vi "testingauto2.vi"() -> ()   [LabVIEW 2014]
uses:
  <vilib>/vision/NI_Vision_Development_Module.lvlib
  <instrlib>/KD Scientific 2XX Series/KD Scientific 2XX Series.lvlib
panel:
  in  "stop 3":bool
  in  "Initial Pressure":dbl[](array[numeric])
  in  "Number of Cycles":i32
  in  "Min Pressure":dbl
  in  "Max Pressure":dbl
  out "Status":T1
  in  "stop 2":bool
  out "Delivered Volume":dbl
  out "Units":string
  in  "Baud Rate (9600)":u32(ring)=9600 items=["300"=300, "1200"=1200, "2400"=2400, "4800"=4800, "9600"=9600]
  in  "Withdrawal Settings":T2={"Flow Rate (5)"=5.0, "Volume (10)"=10.0, "Volume Units (ml)"=enum."milliliters (ml)", "Rate Units (ml/min.)"=enum."milliliters per minute (ml/min.)"} {"Volume (10)" format="%#.3g"}
  in  "Diameter (8.75 mm)":dbl=8.75
  in  "Infusion Settings":T2={"Flow Rate (5)"=5.0, "Volume (10)"=10.0, "Volume Units (ml)"=enum."milliliters (ml)", "Rate Units (ml/min.)"=enum."milliliters per minute (ml/min.)"}
  in  "Address (0)":i32 format="%0.0f"
  in  "error in (no error)":errorcluster
  in  "VISA resource name":refnum<visa-resource-name>="COM1"
  in  "stop":bool
  out "Image":T3(plugin-control)
  out "Particle Measurements (Pixels) (Particle Analysis 1)":dbl[][](array[numeric]) format="%.2f"
  out "subarray":dbl[](array[numeric])
  out "The diameter":dbl[](array[numeric])
  in  "stop (F)":bool
  out "Data from Transducer":dynamicdata(graph) caption="Voltage from Transducer V"
  out "Voltage from pressure transducer":dbl[](array[numeric])
  out "Pressure mm Hg":dbl[](graph)
  in  "Calibration factor":dbl[](array[numeric])
  in  "Zero Error":dbl[](array[numeric])
  out "pressure mm Hg":dbl[](array[numeric])
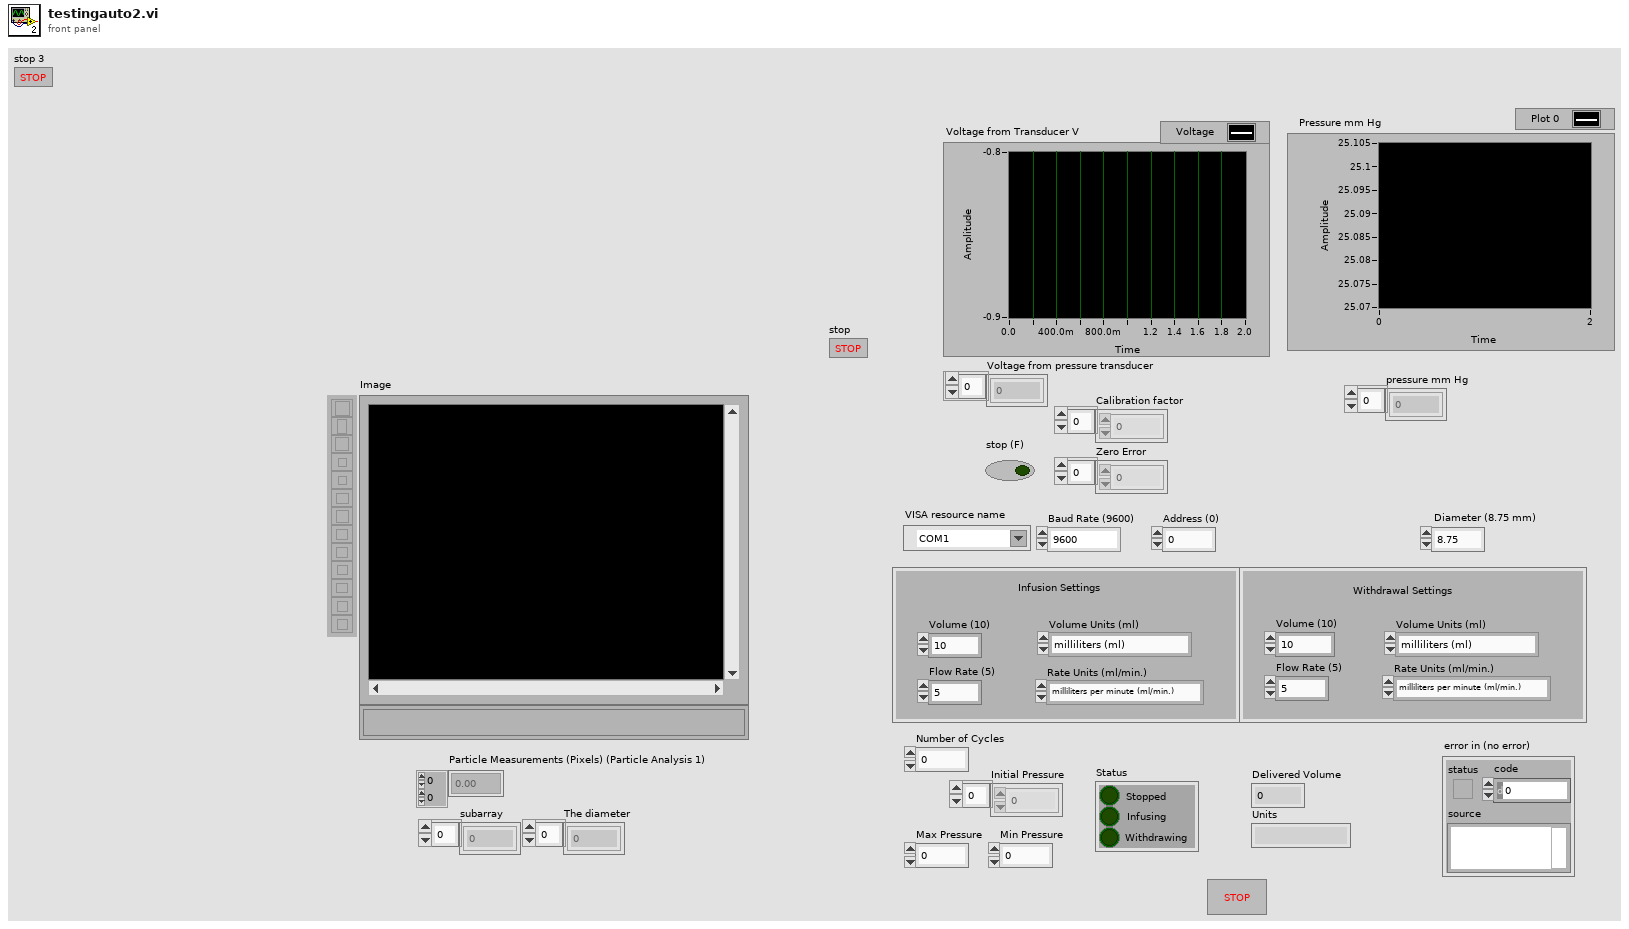
[diagram p1: front panel]
types:
  T1 = cluster{"Stopped":bool, "Infusing":bool, "Withdrawing":bool}
  T2 = cluster{"Flow Rate (5)":dbl, "Volume (10)":dbl, "Volume Units (ml)":enum16{"milliliters (ml)", "microliters (ul)"}, "Rate Units (ml/min.)":enum16{"milliliters per minute (ml/min.)", "milliliters per hour (ml/hr.)", "microliters per minute (ul/min.)", "microliters per hour (ul/hr.)"}}
  T3 = typedef "IMAQ Image.ctl" = refnum<image>
  T4 = typedef "Board Id" = u8
  T5 = typedef "ROI Descriptor" = cluster{"Global Rectangle":i32[], "Contours":cluster{"ID":enum32{"External", "Internal"}, "Type":u32, "Coordinates":i32[]}[]}
  T6 = enum16{"milliliters per minute (ml/min.)", "milliliters per hour (ml/hr.)", "microliters per minute (ul/min.)", "microliters per hour (ul/hr.)"}
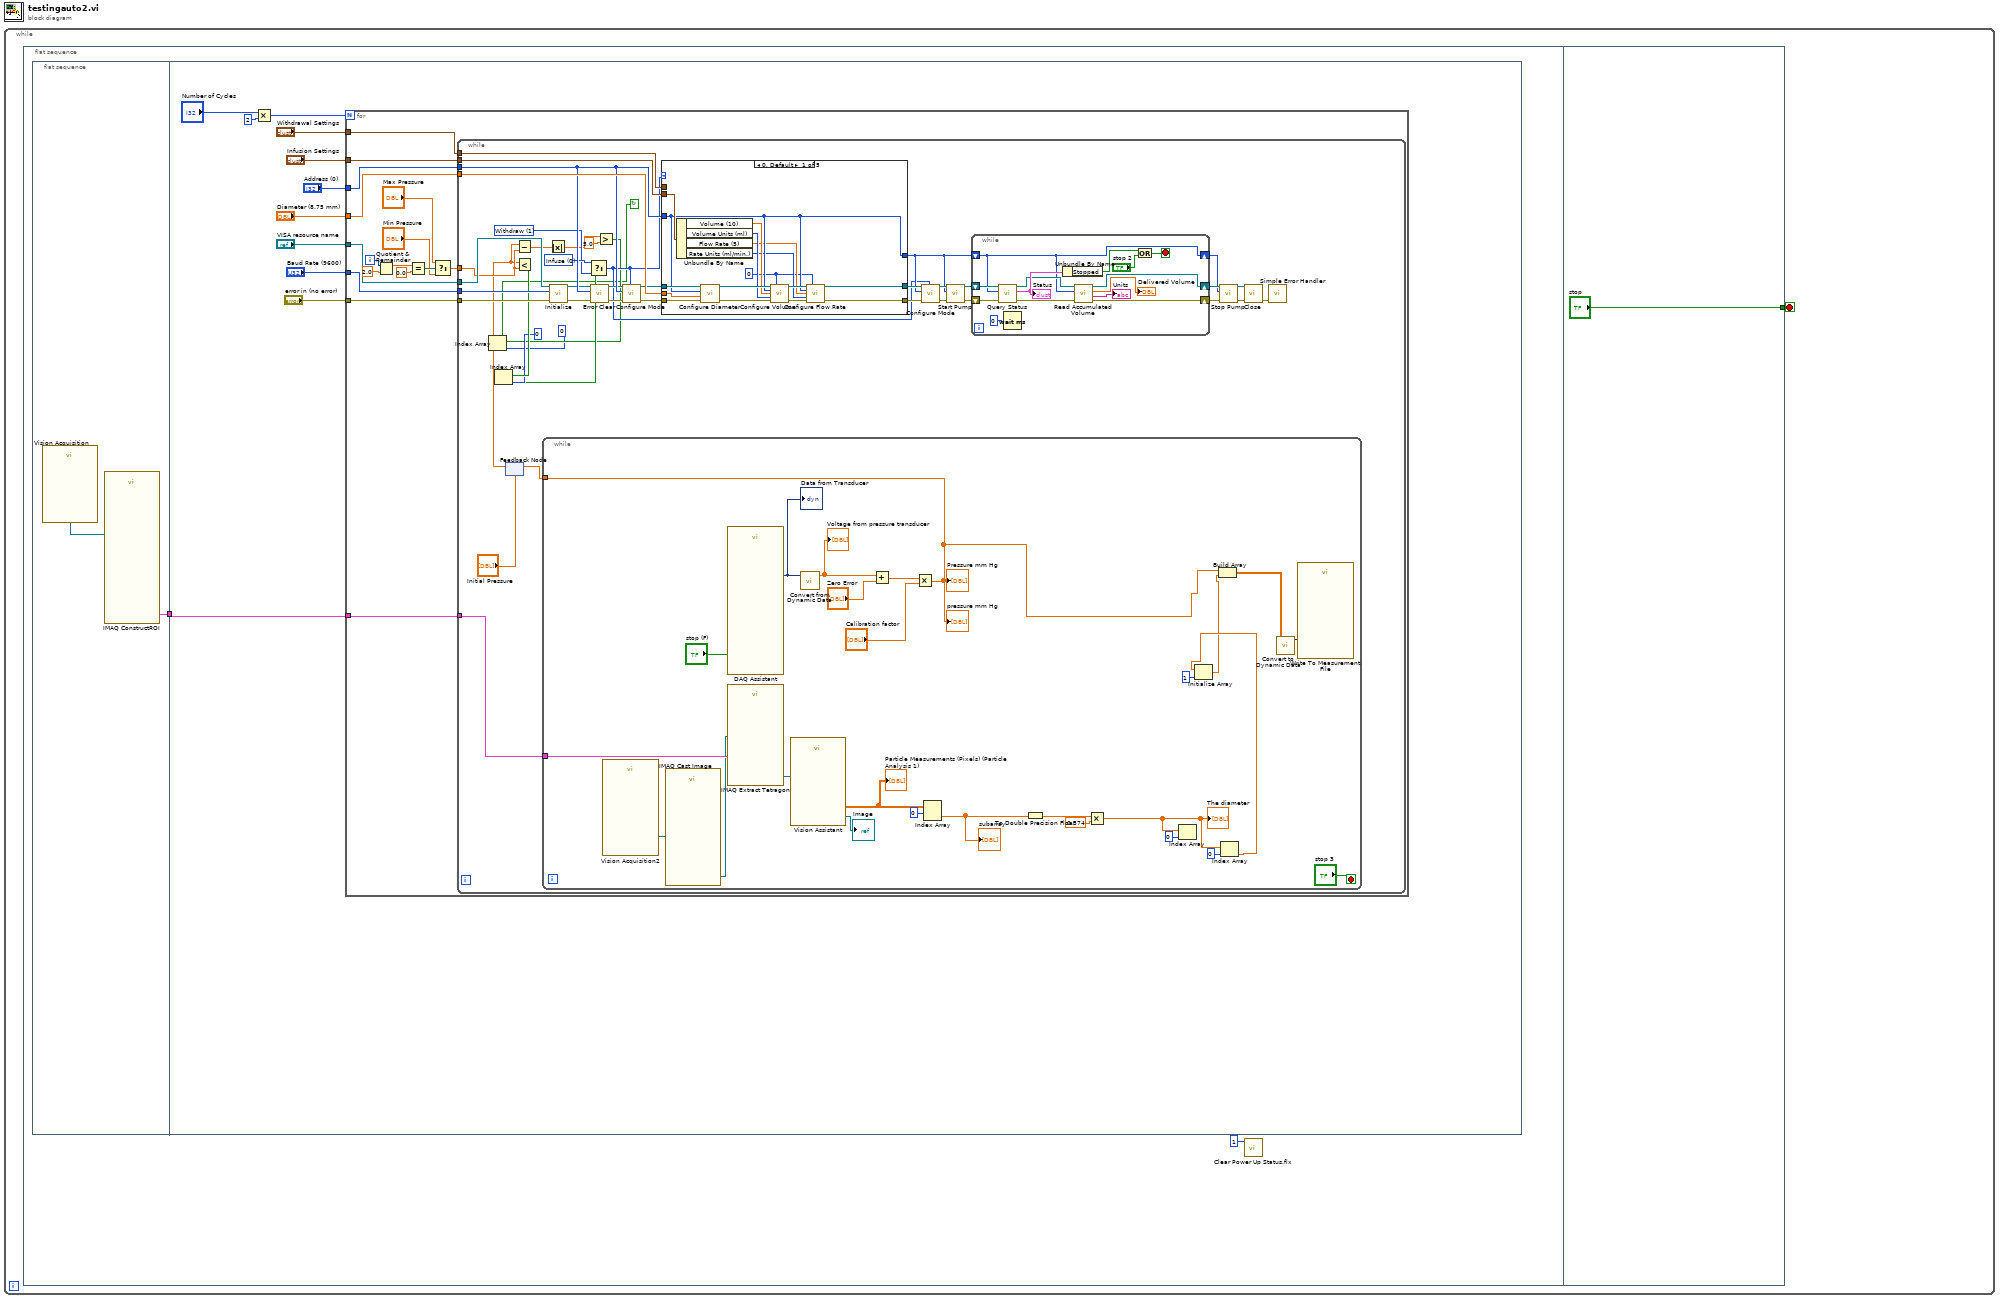
[diagram p0: block diagram]
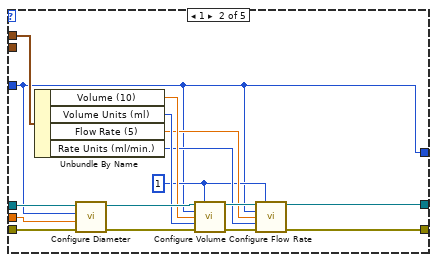
[diagram p2: hidden frame]
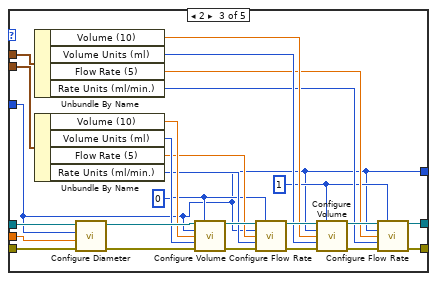
[diagram p3: hidden frame]
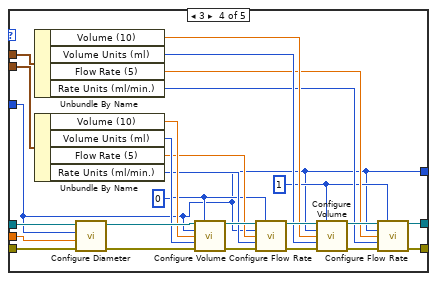
[diagram p4: hidden frame]
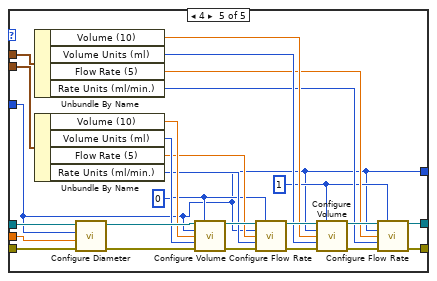
[diagram p5: hidden frame]
diagram:
  n1 = while {
    stop <- w1 stop-if-true
    n2 = flat-sequence {
      tunnel: ["stop"] -> w1
      frame #0 {
        n3 = flat-sequence {
          tunnel: [w4] -> w3
          tunnel: w3 -> [w6]
          frame #0 {
            n4 = call "Vision Acquisition"() -> ("Image Out"=w5:T3)  [unwired: 26 in, 1 out]
            n5 = call "IMAQ ConstructROI"("Image"=w5) -> ("ROI Descriptor Out"=w4:T5)  [unwired: 7 in, 3 out]
          }
          frame #1 {
            n6 = Multiply(x="Number of Cycles", y=2) -> (x*y=w16:i32)
            n7 = for {
              N: w16 -> [_]
              tunnel: "VISA resource name" -> [w32]
              tunnel: "error in (no error)" -> [w31]
              tunnel: "Infusion Settings" -> [w30]
              tunnel: "Withdrawal Settings" -> [w29]
              tunnel: "Diameter (8.75 mm)" -> [w28]
              tunnel: "Baud Rate (9600)" -> [w27]
              tunnel: "Address (0)" -> [w26]
              tunnel: w6 -> [w17]
              i -> [w24]
              n8 = Quotient & Remainder(x=w24, y=2.0) -> (x-y*floor(x/y)=w22:dbl)  [unwired: 1 out]
              n9 = Equal?(x=w22, y=0.0) -> (x = y?=w21:bool)
              n10 = Select(t="Max Pressure", s=w21, f="Min Pressure") -> (s? t:f=w18:dbl)
              n11 = while {
                tunnel: w32 -> [w75]
                tunnel: w31 -> [w74]
                tunnel: w30 -> [w73]
                tunnel: w29 -> [w72]
                tunnel: w28 -> [w71]
                tunnel: w27 -> [w70]
                tunnel: w26 -> [w69]
                tunnel: w18 -> [w46]
                tunnel: w17 -> [w36]
                stop <- w37 continue-if-true
                w48 = u16 1 items=["Withdraw"=1]
                w49 = u16 0 items=["Infuse"] ("Mode (infuse)")
                n12 = feedback #1("Initial Pressure") -> (w34:dbl[])
                n13 = Subtract(x=w34, y=w46) -> (x-y=w45:dbl[])
                n14 = Less?(x=w34, y=w46) -> (x < y?=w42:bool[])
                n15 = Index Array(array=w42, index=0) -> (element=w40:bool)
                n16 = while {
                  tunnel: w36 -> [w84]
                  tunnel: [w81] -> w35
                  stop <- "stop 3" stop-if-true
                  n17 = call "Vision Acquisition2"() -> ("Image Out"=w93:T3)  [unwired: 25 in, 2 out]
                  n18 = call "IMAQ Cast Image"("Image Src"=w93) -> ("Image Dst Out"=w83:T3)  [unwired: 9 in, 1 out]
                  n19 = call "DAQ Assistant"("stop (F)"="stop (F)") -> ("data"=w96:dynamicdata)  [unwired: 15 in, 3 out]
                  "Data from Transducer" <- w96
                  n20 = call-poly "IMAQ Extract Tetragon"("ROI Descriptor"=w84, "Image Src"=w83) -> ("Image Dst Out"=w86:T3)  [unwired: 8 in, 1 out]
                  n21 = call "Vision Assistant"("Image In"=w86) -> ("Image Out"=→"Image":T3, "Particle Measurements (Pixels) (Particle Analysis 1)"=w87:dbl[][])  [unwired: 23 in, 2 out]
                  "Particle Measurements (Pixels) (Particle Analysis 1)" <- w87
                  n22 = call "Convert from Dynamic Data"("Dynamic Data Type"=w96) -> ("Array"=w99:dbl[])  [unwired: 3 in]
                  "Voltage from pressure transducer" <- w99
                  n23 = Add(x=w99, y="Zero Error") -> (x+y=w97:dbl[])
                  n24 = Multiply(x=w97, y="Calibration factor") -> (x*y=w81:dbl[])
                  "Pressure mm Hg" <- w81
                  "pressure mm Hg" <- w81
                  n25 = Index Array(array=w87, index (row)=0) -> (element=w89:dbl[])  [unwired: 1 in]
                  "subarray" <- w89
                  n26 = To Double Precision Float(number=w89) -> (double precision float=w90:dbl[])
                  n27 = Multiply(x=w90, y=0.374) -> (x*y=w95:dbl[])
                  "The diameter" <- w95
                  n28 = Index Array(array=w95, index=0) -> ()  [unwired: 1 out]
                  n29 = Index Array(array=w95, index=0) -> (element=w80:dbl)
                  n30 = Initialize Array(w80, 1 ("dimension size")) -> (w79:dbl[])
                  n31 = Build Array(w81, w79) -> (w78:dbl[][])
                  n32 = call "Convert to Dynamic Data"("2D Array"=w78) -> ("Dynamic Data Type"=w77:dynamicdata)  [unwired: 3 in]
                  n33 = call "Write To Measurement File"("Signals"=w77) -> ()  [unwired: 16 in, 3 out]
                }
                n34 = feedback-in #1(w35) -> ()
                n35 = Absolute Value(x=w45) -> (abs(x)=w44:dbl[])
                n36 = call <instrlib>:"Initialize.vi"("error in (no error)"=w74, "Baud Rate (9600)"=w70, "VISA resource name"=w75) -> ("error out"=w51:errorcluster, "VISA resource name out"=w50:refnum<visa-resource-name>)  [unwired: 7 in]
                n37 = Select(t=w49, s=w40, f=w48) -> (s? t:f=w47:u16)
                n38 = call <instrlib>:"Error Clear.vi"("error in (no error)"=w51, "Address (0)"=w69, "VISA resource name"=w50) -> ("error out"=w52:errorcluster, "VISA resource name out"=w53:refnum<visa-resource-name>)  [unwired: 6 in, 1 out]
                n39 = Greater?(x=w44, y=5.0) -> (0:w39:bool[])
                n40 = Index Array(array=w39, index=0) -> (element=w37:bool)
                n41 = call <instrlib>:"Configure Mode.vi"("Mode (infuse)"=w47, "error in (no error)"=w52, "Address (0)"=w69, "VISA resource name"=w53) -> ("error out"=w55:errorcluster, "VISA resource name out"=w54:refnum<visa-resource-name>)  [unwired: 6 in]
                n42 = case shown="0, Default" w47 {
                  tunnel: w73 -> [w111 _ w159 w185 w211]
                  tunnel: w72 -> [_ w133 w158 w184 w210]
                  tunnel: w54 -> [w117 w132 w157 w183 w209]
                  tunnel: w55 -> [w116 w128 w156 w182 w208]
                  tunnel: w71 -> [w110 w124 w139 w165 w191]
                  tunnel: [w109 w118 w134 w160 w186] -> w56
                  tunnel: w69 -> [w109 w118 w134 w160 w186]
                  tunnel: [w104 w129 w136 w162 w188] -> w60
                  tunnel: [w103 w125 w135 w161 w187] -> w59
                  frame 0, Default {
                    w102 = 0
                    n43 = Unbundle By Name(w111) -> ("Volume (10)"=w108:dbl, "Volume Units (ml)"=w107:enum16{"milliliters (ml)", "microliters (ul)"}, "Flow Rate (5)"=w106:dbl, "Rate Units (ml/min.)"=w105:T6)
                    n44 = call <instrlib>:"Configure Diameter.vi"("error in (no error)"=w116, "Diameter (8.75 mm)"=w110, "Address (0)"=w109, "VISA resource name"=w117) -> ("error out"=w114:errorcluster, "VISA resource name out"=w115:refnum<visa-resource-name>)  [unwired: 6 in]
                    n45 = call <instrlib>:"Configure Volume.vi"("VISA resource name"=w115, "Mode (infuse)"=w102, "Address (0)"=w109, "Volume (100)"=w108, "Units (0: milliliters)"=w107, "error in (no error)"=w114) -> ("VISA resource name out"=w113:refnum<visa-resource-name>, "error out"=w112:errorcluster)  [unwired: 8 in]
                    n46 = call <instrlib>:"Configure Flow Rate.vi"("VISA resource name"=w113, "Mode (infuse)"=w102, "Address (0)"=w109, "Flow Rate (5)"=w106, "Units (0: milliliters per minute)"=w105, "error in (no error)"=w112) -> ("VISA resource name out"=w104:refnum<visa-resource-name>, "error out"=w103:errorcluster)  [unwired: 8 in]
                  }
                  frame 1 {
                    w119 = 1
                    n47 = Unbundle By Name(w133) -> ("Volume (10)"=w123:dbl, "Volume Units (ml)"=w122:enum16{"milliliters (ml)", "microliters (ul)"}, "Flow Rate (5)"=w121:dbl, "Rate Units (ml/min.)"=w120:T6)
                    n48 = call <instrlib>:"Configure Diameter.vi"("error in (no error)"=w128, "Diameter (8.75 mm)"=w124, "Address (0)"=w118, "VISA resource name"=w132) -> ("error out"=w127:errorcluster, "VISA resource name out"=w131:refnum<visa-resource-name>)  [unwired: 6 in]
                    n49 = call <instrlib>:"Configure Volume.vi"("VISA resource name"=w131, "Mode (infuse)"=w119, "Address (0)"=w118, "Volume (100)"=w123, "Units (0: milliliters)"=w122, "error in (no error)"=w127) -> ("VISA resource name out"=w130:refnum<visa-resource-name>, "error out"=w126:errorcluster)  [unwired: 8 in]
                    n50 = call <instrlib>:"Configure Flow Rate.vi"("VISA resource name"=w130, "Mode (infuse)"=w119, "Address (0)"=w118, "Flow Rate (5)"=w121, "Units (0: milliliters per minute)"=w120, "error in (no error)"=w126) -> ("VISA resource name out"=w129:refnum<visa-resource-name>, "error out"=w125:errorcluster)  [unwired: 8 in]
                  }
                  frame 2 {
                    w137 = 1
                    w138 = 0
                    n51 = Unbundle By Name(w158) -> ("Volume (10)"=w143:dbl, "Volume Units (ml)"=w142:enum16{"milliliters (ml)", "microliters (ul)"}, "Flow Rate (5)"=w141:dbl, "Rate Units (ml/min.)"=w140:T6)
                    n52 = Unbundle By Name(w159) -> ("Volume (10)"=w147:dbl, "Volume Units (ml)"=w146:enum16{"milliliters (ml)", "microliters (ul)"}, "Flow Rate (5)"=w145:dbl, "Rate Units (ml/min.)"=w144:T6)
                    n53 = call <instrlib>:"Configure Diameter.vi"("error in (no error)"=w156, "Diameter (8.75 mm)"=w139, "Address (0)"=w134, "VISA resource name"=w157) -> ("error out"=w151:errorcluster, "VISA resource name out"=w155:refnum<visa-resource-name>)  [unwired: 6 in]
                    n54 = call <instrlib>:"Configure Volume.vi"("VISA resource name"=w155, "Mode (infuse)"=w138, "Address (0)"=w134, "Volume (100)"=w147, "Units (0: milliliters)"=w146, "error in (no error)"=w151) -> ("VISA resource name out"=w154:refnum<visa-resource-name>, "error out"=w150:errorcluster)  [unwired: 8 in]
                    n55 = call <instrlib>:"Configure Flow Rate.vi"("VISA resource name"=w154, "Mode (infuse)"=w138, "Address (0)"=w134, "Flow Rate (5)"=w145, "Units (0: milliliters per minute)"=w144, "error in (no error)"=w150) -> ("VISA resource name out"=w153:refnum<visa-resource-name>, "error out"=w149:errorcluster)  [unwired: 8 in]
                    n56 = call <instrlib>:"Configure Volume.vi"("VISA resource name"=w153, "Mode (infuse)"=w137, "Address (0)"=w134, "Volume (100)"=w143, "Units (0: milliliters)"=w142, "error in (no error)"=w149) -> ("VISA resource name out"=w152:refnum<visa-resource-name>, "error out"=w148:errorcluster)  [unwired: 8 in]
                    n57 = call <instrlib>:"Configure Flow Rate.vi"("VISA resource name"=w152, "Mode (infuse)"=w137, "Address (0)"=w134, "Flow Rate (5)"=w141, "Units (0: milliliters per minute)"=w140, "error in (no error)"=w148) -> ("VISA resource name out"=w136:refnum<visa-resource-name>, "error out"=w135:errorcluster)  [unwired: 8 in]
                  }
                  frame 3 {
                    w163 = 1
                    w164 = 0
                    n58 = Unbundle By Name(w184) -> ("Volume (10)"=w169:dbl, "Volume Units (ml)"=w168:enum16{"milliliters (ml)", "microliters (ul)"}, "Flow Rate (5)"=w167:dbl, "Rate Units (ml/min.)"=w166:T6)
                    n59 = Unbundle By Name(w185) -> ("Volume (10)"=w173:dbl, "Volume Units (ml)"=w172:enum16{"milliliters (ml)", "microliters (ul)"}, "Flow Rate (5)"=w171:dbl, "Rate Units (ml/min.)"=w170:T6)
                    n60 = call <instrlib>:"Configure Diameter.vi"("error in (no error)"=w182, "Diameter (8.75 mm)"=w165, "Address (0)"=w160, "VISA resource name"=w183) -> ("error out"=w177:errorcluster, "VISA resource name out"=w181:refnum<visa-resource-name>)  [unwired: 6 in]
                    n61 = call <instrlib>:"Configure Volume.vi"("VISA resource name"=w181, "Mode (infuse)"=w164, "Address (0)"=w160, "Volume (100)"=w173, "Units (0: milliliters)"=w172, "error in (no error)"=w177) -> ("VISA resource name out"=w180:refnum<visa-resource-name>, "error out"=w176:errorcluster)  [unwired: 8 in]
                    n62 = call <instrlib>:"Configure Flow Rate.vi"("VISA resource name"=w180, "Mode (infuse)"=w164, "Address (0)"=w160, "Flow Rate (5)"=w171, "Units (0: milliliters per minute)"=w170, "error in (no error)"=w176) -> ("VISA resource name out"=w179:refnum<visa-resource-name>, "error out"=w175:errorcluster)  [unwired: 8 in]
                    n63 = call <instrlib>:"Configure Volume.vi"("VISA resource name"=w179, "Mode (infuse)"=w163, "Address (0)"=w160, "Volume (100)"=w169, "Units (0: milliliters)"=w168, "error in (no error)"=w175) -> ("VISA resource name out"=w178:refnum<visa-resource-name>, "error out"=w174:errorcluster)  [unwired: 8 in]
                    n64 = call <instrlib>:"Configure Flow Rate.vi"("VISA resource name"=w178, "Mode (infuse)"=w163, "Address (0)"=w160, "Flow Rate (5)"=w167, "Units (0: milliliters per minute)"=w166, "error in (no error)"=w174) -> ("VISA resource name out"=w162:refnum<visa-resource-name>, "error out"=w161:errorcluster)  [unwired: 8 in]
                  }
                  frame 4 {
                    w189 = 1
                    w190 = 0
                    n65 = Unbundle By Name(w210) -> ("Volume (10)"=w195:dbl, "Volume Units (ml)"=w194:enum16{"milliliters (ml)", "microliters (ul)"}, "Flow Rate (5)"=w193:dbl, "Rate Units (ml/min.)"=w192:T6)
                    n66 = Unbundle By Name(w211) -> ("Volume (10)"=w199:dbl, "Volume Units (ml)"=w198:enum16{"milliliters (ml)", "microliters (ul)"}, "Flow Rate (5)"=w197:dbl, "Rate Units (ml/min.)"=w196:T6)
                    n67 = call <instrlib>:"Configure Diameter.vi"("error in (no error)"=w208, "Diameter (8.75 mm)"=w191, "Address (0)"=w186, "VISA resource name"=w209) -> ("error out"=w203:errorcluster, "VISA resource name out"=w207:refnum<visa-resource-name>)  [unwired: 6 in]
                    n68 = call <instrlib>:"Configure Volume.vi"("VISA resource name"=w207, "Mode (infuse)"=w190, "Address (0)"=w186, "Volume (100)"=w199, "Units (0: milliliters)"=w198, "error in (no error)"=w203) -> ("VISA resource name out"=w206:refnum<visa-resource-name>, "error out"=w202:errorcluster)  [unwired: 8 in]
                    n69 = call <instrlib>:"Configure Flow Rate.vi"("VISA resource name"=w206, "Mode (infuse)"=w190, "Address (0)"=w186, "Flow Rate (5)"=w197, "Units (0: milliliters per minute)"=w196, "error in (no error)"=w202) -> ("VISA resource name out"=w205:refnum<visa-resource-name>, "error out"=w201:errorcluster)  [unwired: 8 in]
                    n70 = call <instrlib>:"Configure Volume.vi"("VISA resource name"=w205, "Mode (infuse)"=w189, "Address (0)"=w186, "Volume (100)"=w195, "Units (0: milliliters)"=w194, "error in (no error)"=w201) -> ("VISA resource name out"=w204:refnum<visa-resource-name>, "error out"=w200:errorcluster)  [unwired: 8 in]
                    n71 = call <instrlib>:"Configure Flow Rate.vi"("VISA resource name"=w204, "Mode (infuse)"=w189, "Address (0)"=w186, "Flow Rate (5)"=w193, "Units (0: milliliters per minute)"=w192, "error in (no error)"=w200) -> ("VISA resource name out"=w188:refnum<visa-resource-name>, "error out"=w187:errorcluster)  [unwired: 8 in]
                  }
                }
                n72 = call <instrlib>:"Configure Mode.vi"("Mode (infuse)"=w47, "error in (no error)"=w59, "Address (0)"=w56, "VISA resource name"=w60) -> ("error out"=w57:errorcluster, "VISA resource name out"=w58:refnum<visa-resource-name>)  [unwired: 6 in]
                n73 = call <instrlib>:"Start Pump.vi"("error in (no error)"=w57, "Address (0)"=w56, "VISA resource name"=w58) -> ("error out"=w67:errorcluster, "VISA resource name out"=w68:refnum<visa-resource-name>)  [unwired: 7 in]
                n74 = while {
                  shift-right: [w214] -> w64
                  shift-left: w56 -> [w214]
                  shift-right: [w216] -> w66
                  shift-left: w68 -> [w222]
                  shift-right: [w215] -> w65
                  shift-left: w67 -> [w223]
                  stop <- w220 stop-if-true
                  n75 = call <instrlib>:"Query Status.vi"("error in (no error)"=w223, "Address (0)"=w214, "VISA resource name"=w222) -> ("error out"=w225:errorcluster, "Status"=w221:T1, "VISA resource name out"=w217:refnum<visa-resource-name>)  [unwired: 6 in]
                  "Status" <- w221
                  n76 = Wait (ms)(milliseconds to wait=u32 0) -> ()  [unwired: 1 out]
                  n77 = Unbundle By Name(w221) -> ("Stopped"=w219:bool)
                  n78 = call <instrlib>:"Read Accumulated Volume.vi"("error in (no error)"=w225, "Address (0)"=w214, "VISA resource name"=w217) -> ("error out"=w215:errorcluster, "Units"=→"Units":string, "Delivered Volume"=→"Delivered Volume":dbl, "VISA resource name out"=w216:refnum<visa-resource-name>)  [unwired: 5 in]
                  n79 = Or(x=w219, y="stop 2") -> (x .or. y?=w220:bool)
                }
                n80 = call <instrlib>:"Stop Pump.vi"("error in (no error)"=w65, "Address (0)"=w64, "VISA resource name"=w66) -> ("error out"=w62:errorcluster, "VISA resource name out"=w61:refnum<visa-resource-name>)  [unwired: 7 in]
                n81 = call <instrlib>:"Close.vi"("error in (no error)"=w62, "VISA resource name"=w61) -> ("error out"=w63:errorcluster)  [unwired: 9 in]
                n82 = call <vilib>:"Simple Error Handler.vi"("error in (no error)"=w63) -> ()  [unwired: 4 in, 5 out]
              }
            }
          }
        }
        n83 = call <vilib>:"Clear Power Up Status.flx"("Board ID"=T4 1) -> ()  [unwired: 6 in, 2 out]
      }
      frame #1 {
      }
    }
  }
